vi "CalculateTicks.vi"(10 "Distance (in)":dbl, 11 "Motor Settings":T1) -> (3 "Ticks":dbl)   [LabVIEW 2015]
uses:
  Advanced Drive VIs/Drive Motor Settings.ctl
panel:
  out "Motor Rotations":dbl
  out "Wheel Rotations":dbl
  out "Wheel perimeter":dbl
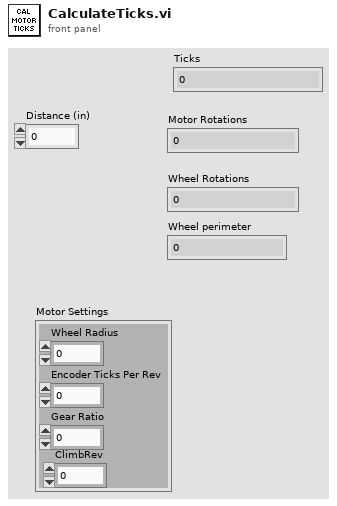
[diagram p1: front panel]
types:
  T1 = typedef "Drive Motor Settings.ctl" = cluster{"Wheel Radius":dbl, "Encoder Ticks Per Rev":dbl, "Gear Ratio":dbl, "ClimbRev":dbl}
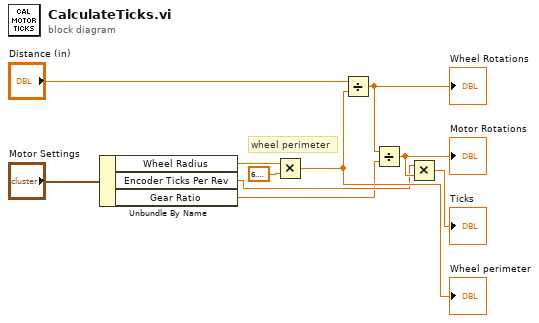
[diagram p0: block diagram]
diagram:
  # "wheel perimeter"
  n1 = Unbundle By Name("Motor Settings") -> ("Wheel Radius"=w4:dbl, "Encoder Ticks Per Rev"=w3:dbl, "Gear Ratio"=w2:dbl)
  n2 = Multiply(x=w4, y=6.283185307179586) -> (x*y=w6:dbl)
  "Wheel perimeter" <- w6
  n3 = Divide(x="Distance (in)", y=w6) -> (x/y=w9:dbl)
  "Wheel Rotations" <- w9
  n4 = Divide(x=w9, y=w2) -> (x/y=w7:dbl)
  "Motor Rotations" <- w7
  n5 = Multiply(x=w3, y=w7) -> (x*y=→"Ticks":dbl)
